vi "Do Core.vi"(8 "error in (no error)":errorcluster, 9 "Actor in":refnum<class "Actor.lvclass">, 11 "Reply Message":refnum<class "Read NowTime Msg.lvclass">) -> (0 "error out":errorcluster, 1 "Actor out":refnum<class "Actor.lvclass">, 2 "Reply":variant)   [LabVIEW 2014, in "RealWorkActor.lvlib" / "Read NowTime Msg.lvclass"]
doc: "(<B>Filename</B>: Actor Framework.lvlib:Reply Msg.lvclass:Do Core.vi)\n\nDefines what an actor does when it receives <B>Reply Message</B>. This method also defines the <B>Reply</B> that is returned to the actor that sent <B>Reply Message</B>.\n\nBy default, this method does nothing, and <B>Reply</B> is the ancestor Message class. A child class must override this method to define behavior and specify a child of the Message class to return in the <B>Reply</B> output."
uses:
  Read NowTime Msg.lvclass
  RealWorkActor/RealWorkActor.lvclass
  <vilib>/ActorFramework/Actor/Actor.lvclass
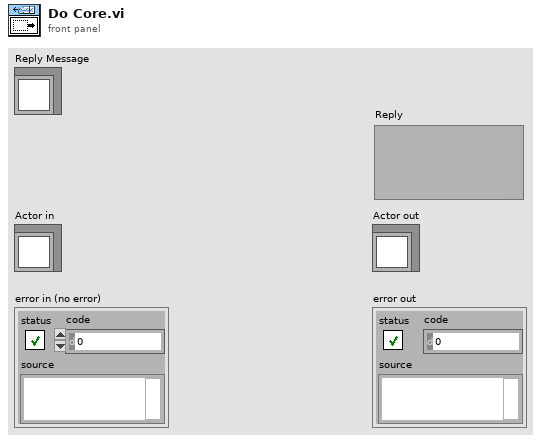
[diagram p1: front panel]
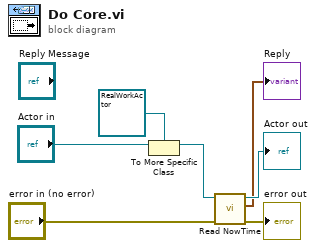
[diagram p0: block diagram]
diagram:
  n1 = To More Specific Class(target class=refnum<class "RealWorkActor.lvclass"> refnum ("RealWorkActor.lvlib:RealWorkActor.lvclass"), reference="Actor in") -> (specific class reference=w2:refnum<class "RealWorkActor.lvclass">)  [unwired: 1 in, 1 out]
  n2 = call "Read NowTime.vi"("error in (no error)"="error in (no error)", "RealWorkActor in"=w2) -> ("error out"=→"error out":errorcluster, "NowTime"=→"Reply":timestamp, "RealWorkActor out"=→"Actor out":refnum<class "RealWorkActor.lvclass">)  [unwired: 7 in]
